vi "GetTemplate.vi"(8 "error in (no error)":errorcluster, 11 "OneOfTemplate in":refnum<class "nidaqmx_grpc_CreateDOChanRequest_line_grouping_enum.lvclass">) -> (0 "error out":errorcluster, 2 "Get_Val":i32, 3 "OneOfTemplate out":refnum<class "nidaqmx_grpc_CreateDOChanRequest_line_grouping_enum.lvclass">)   [LabVIEW 2021, in "NI_DAQmx_client.lvlib" / "nidaqmx_grpc_CreateDOChanRequest_line_grouping_enum.lvclass"]
uses:
  nidaqmx_grpc_CreateDOChanRequest_line_grouping_enum.lvclass
  nidaqmx_grpc_CreateDOChanRequest_line_grouping_enum.lvclass/nidaqmx_grpc_CreateDOChanRequest_line_grouping_enum.ctl
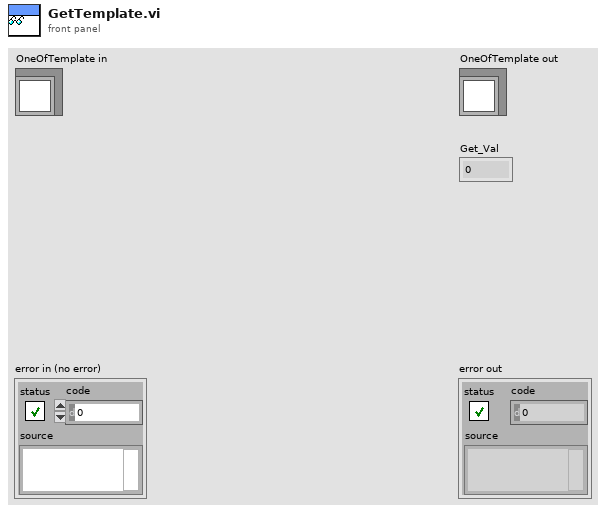
[diagram p1: front panel]
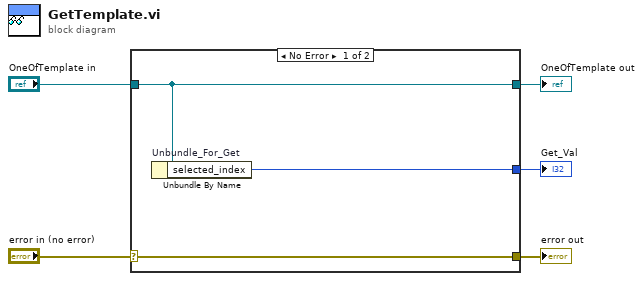
[diagram p0: block diagram]
diagram:
  n1 = case shown="No Error" "error in (no error)" {
    selector: "error in (no error)" -> [w8 w9]
    tunnel: [w8 w9] -> w4
    tunnel: [w7 w10] -> w2
    tunnel: "OneOfTemplate in" -> [w7 w10]
    tunnel: [w6 _] -> w1
    frame No Error {
      n2 = Unbundle By Name "Unbundle_For_Get"(w7) -> ("selected_index"=w6:i32)
    }
    frame Error {
    }
  }
  "error out" <- w4
  "OneOfTemplate out" <- w2
  "Get_Val" <- w1
